vi "Test all Data Types in Variant.vi"() -> ()   [LabVIEW 2017]
uses:
  95ab98eb-4936-488b-be02-d4752316b10a.vi
  4a70d5b1-c23f-48dd-b608-4a2b1e28297d.vi
  Variant to JSON Text.vi
  JSON text to Variant.vi
  <vilib>/addons/_JKI Toolkits/Caraya/classes/Test/Test.lvclass
  <vilib>/addons/_JKI Toolkits/Caraya/classes/Assert/Assert.lvclass
  <vilib>/JDP Science/JDP Science Common Utilities/JDP Utility.lvlib
  <vilib>/Utility/Data Type/NI_Data Type.lvlib
panel:
  out "Variant in":variant
  out "error out":errorcluster
  out "<JSON>":string
  out "Variant out":variant
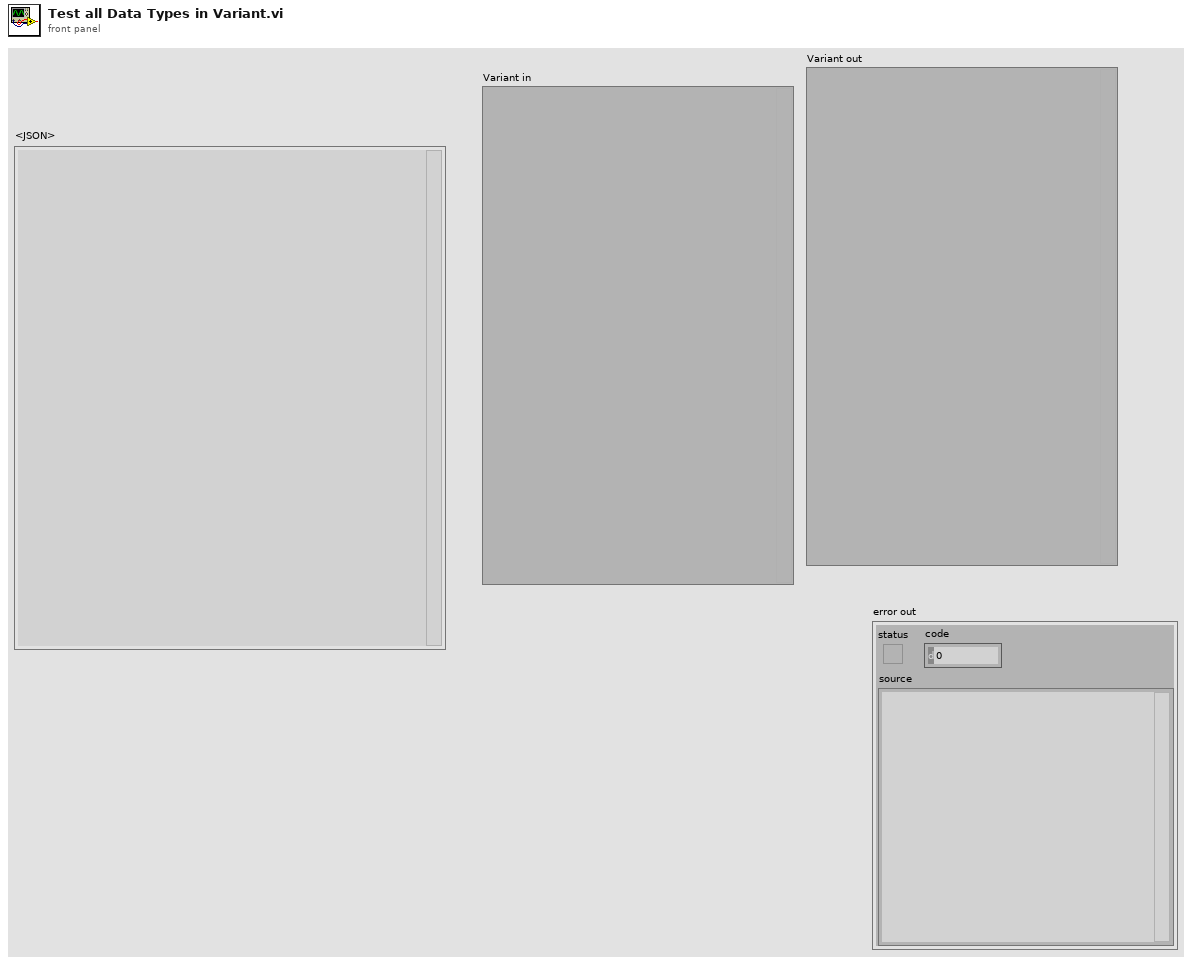
[diagram p1: front panel]
types:
  T1 = cluster{"Number":i32, "String":string, "Timestamp":timestamp, "Queue refnum":refnum<queue>, "VISA resource name":refnum<visa-resource-name>, "occurrence":refnum<k4>, "Boolean":bool, "Enum":enum16{"Enum 1", "Enum 22", "Enum 333"}, "DBL":dbl, "Enum Array":enum16{"Enum 1", "Enum 22", "Enum 333"}[], "Timestamp array":timestamp[], "DBL Array":dbl[], "String Array":string[], "fixed-point":fxp<+/-,32,16>, "fixed-point Array":fxp<+/-,32,16>[], "Path":path}
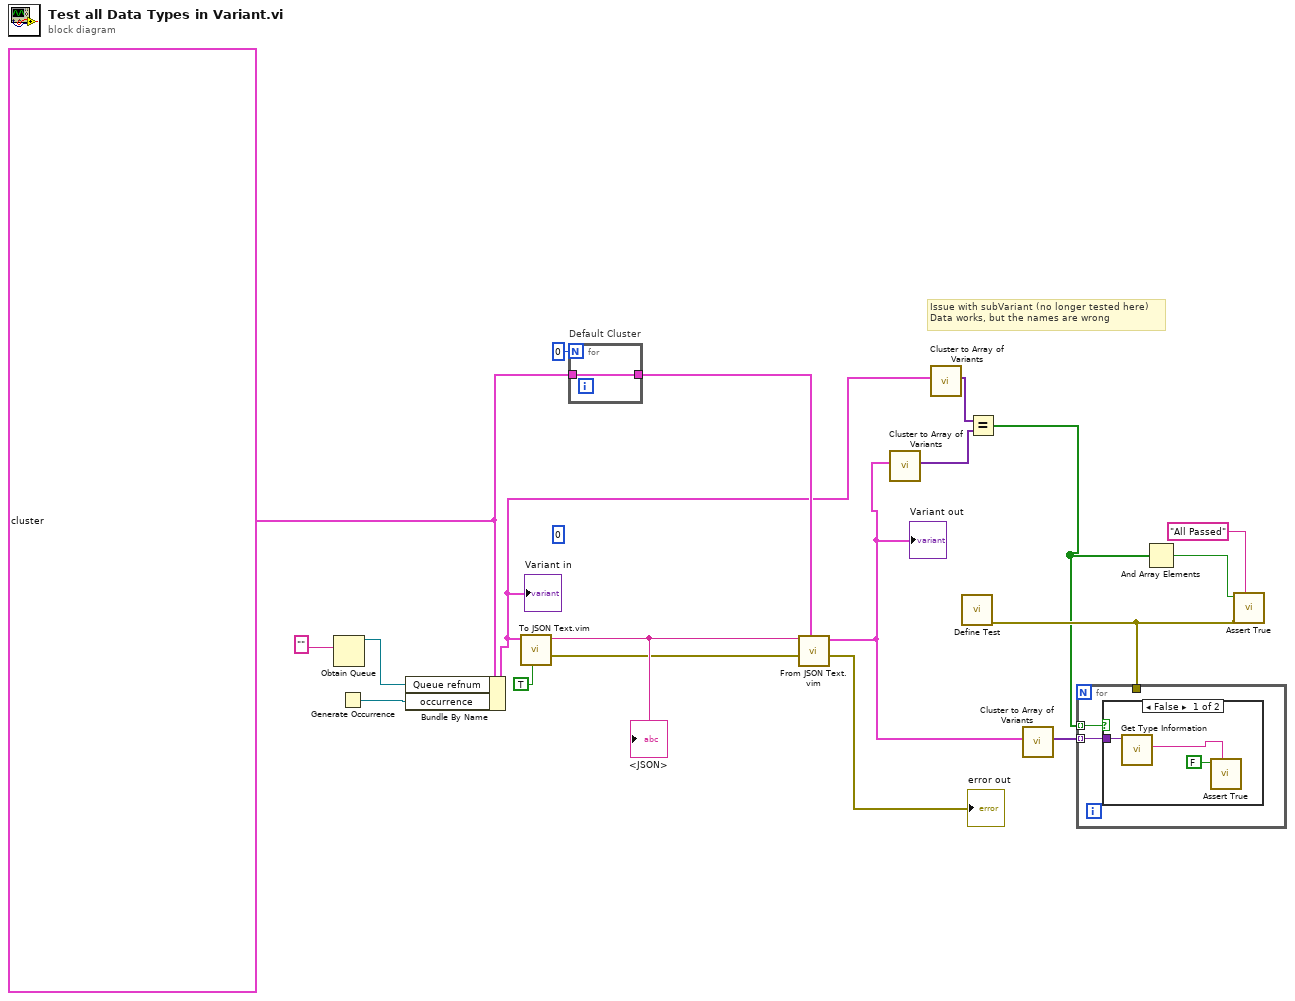
[diagram p0: block diagram]
diagram:
  (unwired) 0
  w14 = T1 {"Number"=1234, "String"="Hello", "Timestamp"=timestamp(3557316526.864 s since 1904-01-01), "Queue refnum"=refnum, "VISA resource name"="COM3", "occurrence"=refnum, "Boolean"=TRUE, "Enum"=enum."Enum 22", "DBL"=1234.56789012345, "Enum Array"=[enum."Enum 333", enum."Enum 22", enum."Enum 1"], "Timestamp array"=[timestamp(3557316526.864 s since 1904-01-01), timestamp(3538916926.864 s since 1904-01-01), timestamp(3588852526.864 s since 1904-01-01)], "DBL Array"=[1234.5678901234, 1234.5678901234, 1.3245235436654], "String Array"=["Hello", "There", "||¬¬¬¬¬"], "fixed-point"=32767.899993896484, "fixed-point Array"=[32767.899993896484, 0.0010223388671875, 4234.756866455078], "Path"=path "C:/JSONtext"}
  # "Issue with subVariant (no longer tested here)\nData works, but the names are wrong"
  n1 = Obtain Queue(element data type="") -> (queue out=w17:refnum<queue>)  [unwired: 4 in, 2 out]
  n2 = Generate Occurrence() -> (w15:refnum<k4>)
  n3 = Bundle By Name(cluster=w14, "Queue refnum"=w17, "occurrence"=w15) -> (w1:T1)
  "Variant in" <- w1
  n4 = call "To JSON Text.vim"("Pretty Print?"=TRUE, "Anything"=w1) -> ("error out"=w10:errorcluster, "<JSON>"=w19:string)  [unwired: 8 in]
  "<JSON>" <- w19
  n5 = for "Default Cluster" {
    N: 0 -> [_]
    tunnel: w14 -> [w20]
    tunnel: [w20] -> w13
  }
  n6 = call "From JSON Text.vim"("Data Type and Default Value"=w13, "error in (no error)"=w10, "JSON"=w19) -> ("error out"=→"error out":errorcluster, "Data out"=w5:T1)  [unwired: 7 in]
  "Variant out" <- w5
  n7 = call <vilib>:"Cluster to Array of Variants.vi"("Cluster"=w5) -> ("Array of Cluster Elements"=w4:variant[])  [unwired: 10 in]
  n8 = call <vilib>:"Cluster to Array of Variants.vi"("Cluster"=w1) -> ("Array of Cluster Elements"=w3:variant[])  [unwired: 10 in]
  n9 = call <vilib>:"Define Test.vi"() -> ("error out"=w7:errorcluster)  [unwired: 11 in]
  n10 = Equal?(x=w3, y=w4) -> (x = y?=w2:bool[])
  n11 = call <vilib>:"Cluster to Array of Variants.vi"("Cluster"=w5) -> ("Array of Cluster Elements"=w8:variant[])  [unwired: 10 in]
  n12 = for {
    tunnel: w2 -> [w22] mode=indexing
    tunnel: w8 -> [w21] mode=indexing
    tunnel: w7 -> [_]
    n13 = case shown="False" w22 {
      tunnel: w21 -> [w25 _]
      frame False {
        n14 = call <vilib>:"Get Type Information.vi"("Variant"=w25) -> ("Name"=w24:string)  [unwired: 6 in, 4 out]
        n15 = call <vilib>:"Assert True.vi"("Label"=w24, "True?"=FALSE) -> ()  [unwired: 9 in, 1 out]
      }
      frame True {
      }
    }
  }
  n16 = And Array Elements(Boolean array=w2) -> (logical AND=w6:bool)
  n17 = call <vilib>:"Assert True.vi"("Label"="All Passed", "error in (no error)"=w7, "True?"=w6) -> ()  [unwired: 8 in, 1 out]
